vi "LT_get_param.vi"(6 "param_index":u16 step=1, 7 "param_number":u16=1 min=1 step=1, 8 "error in":errorcluster, 10 "dev_param_in":T1={"Length of data block (14)"=14, "Converter address (0)"=0, "Converter type\n(180: Turbovac 350/450 i)"=180, "PZD1 STW, ZSW (0)"=0, "PZD2 HSW, HIW (0)"=0} {"Converter type\n(180: Turbovac 350/450 i)" items=["Turbovac 350/450 i"=180, "Turbovac 350/450 i with optional interface"=181, "Turbovac 350/450 iX"=182, "Turbovac  90/250 i"=190, "Turbovac  90/250 with optional interface"=191, "Turbovac  90/250 iX"=192, "Turbovac  850/950 i"=195, "Turbovac  850/950 i with optional interface"=196, "Turbovac  850/950 iX"=197, "Turbovac 1350/1450 i"=185, "Turbovac 1350/1450 i with optional interface"=186, "Turbovac 1350/1450 iX"=187]; "Length of data block (14)" items=["14"=14, "22"=22]}, 11 "VISA in":refnum<visa-resource-name>="COM43") -> (0 "error out":errorcluster, 2 "dev_param_out":T3={"Length of data block"=14, "Converter address"=0, "Converter type"=180, "PZD1"=0, "PZD2"=0} {"Converter type" items=["Turbovac 350/450 i"=180, "Turbovac 350/450 i with optional interface"=181, "Turbovac 350/450 iX"=182, "Turbovac  90/250 i"=190, "Turbovac  90/250 with optional interface"=191, "Turbovac  90/250 iX"=192, "Turbovac  850/950 i"=195, "Turbovac  850/950 i with optional interface"=196, "Turbovac  850/950 iX"=197, "Turbovac 1350/1450 i"=185, "Turbovac 1350/1450 i with optional interface"=186, "Turbovac 1350/1450 iX"=187]; "Length of data block" items=["14"=14, "22"=22]}, 3 "VISA out":refnum<visa-resource-name>, 4 "PWE":i32)   [LabVIEW 2019]
doc: "Example VI to demonstrate the use of the Oerlikon Leybold TMP driver."
uses:
  <instrlib>/Leybold TURBOVAC/Public/Ctl/Device Parameters Indicator.ctl
  <instrlib>/Leybold TURBOVAC/Public/Ctl/Converter Type Indicator.ctl
  <instrlib>/Leybold TURBOVAC/Public/Ctl/Device Parameters Control.ctl
  <instrlib>/Leybold TURBOVAC/Public/Ctl/Converter Type Control.ctl
  <instrlib>/Leybold TURBOVAC/Leybold TURBOVAC.lvlib
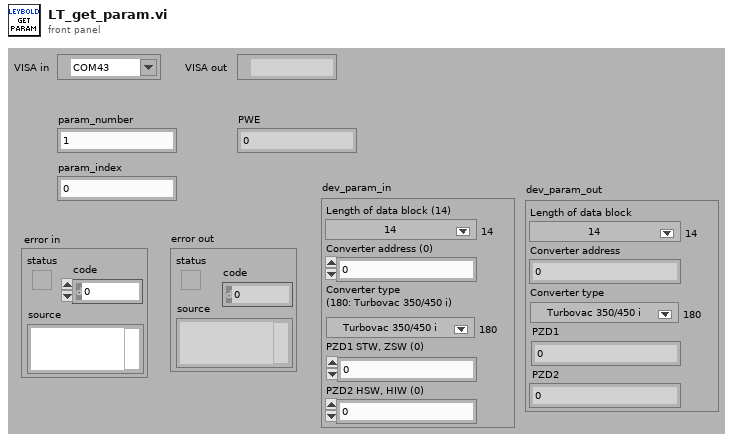
[diagram p1: front panel]
types:
  T1 = typedef "Leybold TURBOVAC.lvlib/Device Parameters Control.ctl" = cluster{"Length of data block (14)":u8, "Converter address (0)":u8, "Converter type\n(180: Turbovac 350/450 i)":T2, "PZD1 STW, ZSW (0)":u16, "PZD2 HSW, HIW (0)":u16}
  T2 = typedef "Leybold TURBOVAC.lvlib/Converter Type Control.ctl" = u16
  T3 = typedef "Leybold TURBOVAC.lvlib/Device Parameters Indicator.ctl" = cluster{"Length of data block":u8, "Converter address":u8, "Converter type":T4, "PZD1":u16, "PZD2":u16}
  T4 = typedef "Leybold TURBOVAC.lvlib/Converter Type Indicator.ctl" = u16
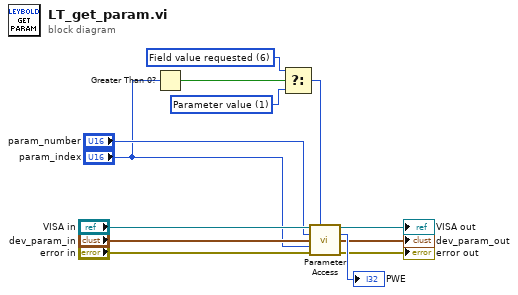
[diagram p0: block diagram]
diagram:
  w2 = u8 6 items=["Do nothing"=0, "Parameter value"=1, "Write 16 bit value"=2, "Write 32 bit value"=3, "Field value requested"=6, "Write 16 bit field value"=7, "Write 32 bit field value"=8, "Request No. of field elements"=9] ("Type of parameter access (1: Parameter value)")
  w3 = u8 1 items=["Do nothing"=0, "Parameter value"=1, "Write 16 bit value"=2, "Write 32 bit value"=3, "Field value requested"=6, "Write 16 bit field value"=7, "Write 32 bit field value"=8, "Request No. of field elements"=9] ("Type of parameter access (1: Parameter value)")
  n1 = Greater Than 0?(x="param_index") -> (x > 0?=w4:bool)
  n2 = Select(t=w2, s=w4, f=w3) -> (s? t:f=w1:u8)
  n3 = call <instrlib>:"Parameter Access.vi"("VISA resource name"="VISA in", "Type of parameter access (1: Parameter value)"=w1, "PKE-PM No. (1)"="param_number", "Device parameters"="dev_param_in", "Index (0)"="param_index", "error in (no error)"="error in") -> ("VISA resource name out"=→"VISA out":refnum<visa-resource-name>, "PWE out"=→"PWE":i32, "Device parameters out"=→"dev_param_out":T3, "error out"=→"error out":errorcluster)  [unwired: 6 in]
